vi "cam3 analyse.vi"() -> (0 "G3 chiffre":string, 1 "Y4 chiffre":string, 2 "Y7 chiffre":string, 3 "R2 chiffre":string, 4 "R7 chiffre":string, 5 "G6 chiffre":string, 7 "G9 chiffre":string, 9 "Y1 chiffre":string, 11 "Y2 chiffre":string, 12 "Y3 chiffre":string, 13 "R1 chiffre":string, 14 "R4 chiffre":string)   [LabVIEW 2019]
uses:
  <vilib>/vision/Classification.llb/IMAQ Classifier Read Options.ctl
  <vilib>/vision/NI_Vision_Development_Module.lvlib
panel:
  in  "R7":T1={"Global Rectangle"=[0, 0, 1279, 959], "Contours"=[{"ID"=enum."External", "Type"=3, "Coordinates"=[0, 0, 1279, 959]}]} {"Contours"."Type" items=["No Selection", "Point", "Line", "Rectangle", "Oval", "Polygon", "Freehand Region", "Annulus", "Unused2", "Unused3", "Broken Line", "Freehand Line", "Rotated Rectangle"]}
  out "R7":string[](array[string])
  in  "Y4   3":T1={"Global Rectangle"=[0, 0, 1279, 959], "Contours"=[{"ID"=enum."External", "Type"=3, "Coordinates"=[0, 0, 1279, 959]}]} {"Contours"."Type" items=["No Selection", "Point", "Line", "Rectangle", "Oval", "Polygon", "Freehand Region", "Annulus", "Unused2", "Unused3", "Broken Line", "Freehand Line", "Rotated Rectangle"]}
  out "Y4 2":string[](array[string])
  in  "error in":errorcluster
  out "Coordinates":i32[](array[numeric])
  in  "R4":T1={"Global Rectangle"=[0, 0, 1279, 959], "Contours"=[{"ID"=enum."External", "Type"=3, "Coordinates"=[0, 0, 1279, 959]}]} {"Contours"."Type" items=["No Selection", "Point", "Line", "Rectangle", "Oval", "Polygon", "Freehand Region", "Annulus", "Unused2", "Unused3", "Broken Line", "Freehand Line", "Rotated Rectangle"]}
  out "R4":string[](array[string])
  in  "R2":T1={"Global Rectangle"=[0, 0, 1279, 959], "Contours"=[{"ID"=enum."External", "Type"=3, "Coordinates"=[0, 0, 1279, 959]}]} {"Contours"."Type" items=["No Selection", "Point", "Line", "Rectangle", "Oval", "Polygon", "Freehand Region", "Annulus", "Unused2", "Unused3", "Broken Line", "Freehand Line", "Rotated Rectangle"]}
  out "R2":string[](array[string])
  in  "R1":T1={"Global Rectangle"=[0, 0, 1279, 959], "Contours"=[{"ID"=enum."External", "Type"=3, "Coordinates"=[0, 0, 1279, 959]}]} {"Contours"."Type" items=["No Selection", "Point", "Line", "Rectangle", "Oval", "Polygon", "Freehand Region", "Annulus", "Unused2", "Unused3", "Broken Line", "Freehand Line", "Rotated Rectangle"]}
  out "R1":string[](array[string])
  in  "Y7":T1={"Global Rectangle"=[0, 0, 1279, 959], "Contours"=[{"ID"=enum."External", "Type"=3, "Coordinates"=[0, 0, 1279, 959]}]} {"Contours"."Type" items=["No Selection", "Point", "Line", "Rectangle", "Oval", "Polygon", "Freehand Region", "Annulus", "Unused2", "Unused3", "Broken Line", "Freehand Line", "Rotated Rectangle"]}
  out "Y7":string[](array[string])
  in  "Y3":T1={"Global Rectangle"=[0, 0, 1279, 959], "Contours"=[{"ID"=enum."External", "Type"=3, "Coordinates"=[0, 0, 1279, 959]}]} {"Contours"."Type" items=["No Selection", "Point", "Line", "Rectangle", "Oval", "Polygon", "Freehand Region", "Annulus", "Unused2", "Unused3", "Broken Line", "Freehand Line", "Rotated Rectangle"]}
  out "Y3":string[](array[string])
  in  "Y2":T1={"Global Rectangle"=[0, 0, 1279, 959], "Contours"=[{"ID"=enum."External", "Type"=3, "Coordinates"=[0, 0, 1279, 959]}]} {"Contours"."Type" items=["No Selection", "Point", "Line", "Rectangle", "Oval", "Polygon", "Freehand Region", "Annulus", "Unused2", "Unused3", "Broken Line", "Freehand Line", "Rotated Rectangle"]}
  out "Y2":string[](array[string])
  in  "Y1":T1={"Global Rectangle"=[0, 0, 1279, 959], "Contours"=[{"ID"=enum."External", "Type"=3, "Coordinates"=[0, 0, 1279, 959]}]} {"Contours"."Type" items=["No Selection", "Point", "Line", "Rectangle", "Oval", "Polygon", "Freehand Region", "Annulus", "Unused2", "Unused3", "Broken Line", "Freehand Line", "Rotated Rectangle"]}
  out "Y1":string[](array[string])
  in  "G9":T1={"Global Rectangle"=[0, 0, 1279, 959], "Contours"=[{"ID"=enum."External", "Type"=3, "Coordinates"=[0, 0, 1279, 959]}]} {"Contours"."Type" items=["No Selection", "Point", "Line", "Rectangle", "Oval", "Polygon", "Freehand Region", "Annulus", "Unused2", "Unused3", "Broken Line", "Freehand Line", "Rotated Rectangle"]}
  out "G9":string[](array[string])
  in  "G6":T1={"Global Rectangle"=[0, 0, 1279, 959], "Contours"=[{"ID"=enum."External", "Type"=3, "Coordinates"=[0, 0, 1279, 959]}]} {"Contours"."Type" items=["No Selection", "Point", "Line", "Rectangle", "Oval", "Polygon", "Freehand Region", "Annulus", "Unused2", "Unused3", "Broken Line", "Freehand Line", "Rotated Rectangle"]}
  out "G6":string[](array[string])
  in  "G3":T1={"Global Rectangle"=[640, 450, 686, 504], "Contours"=[{"ID"=enum."External", "Type"=3, "Coordinates"=[640, 450, 686, 504]}]} {"Contours"."Type" items=["No Selection", "Point", "Line", "Rectangle", "Oval", "Polygon", "Freehand Region", "Annulus", "Unused2", "Unused3", "Broken Line", "Freehand Line", "Rotated Rectangle"]}
  out "Image Out 2":T2(plugin-control)
  out "G3":string[](array[string])
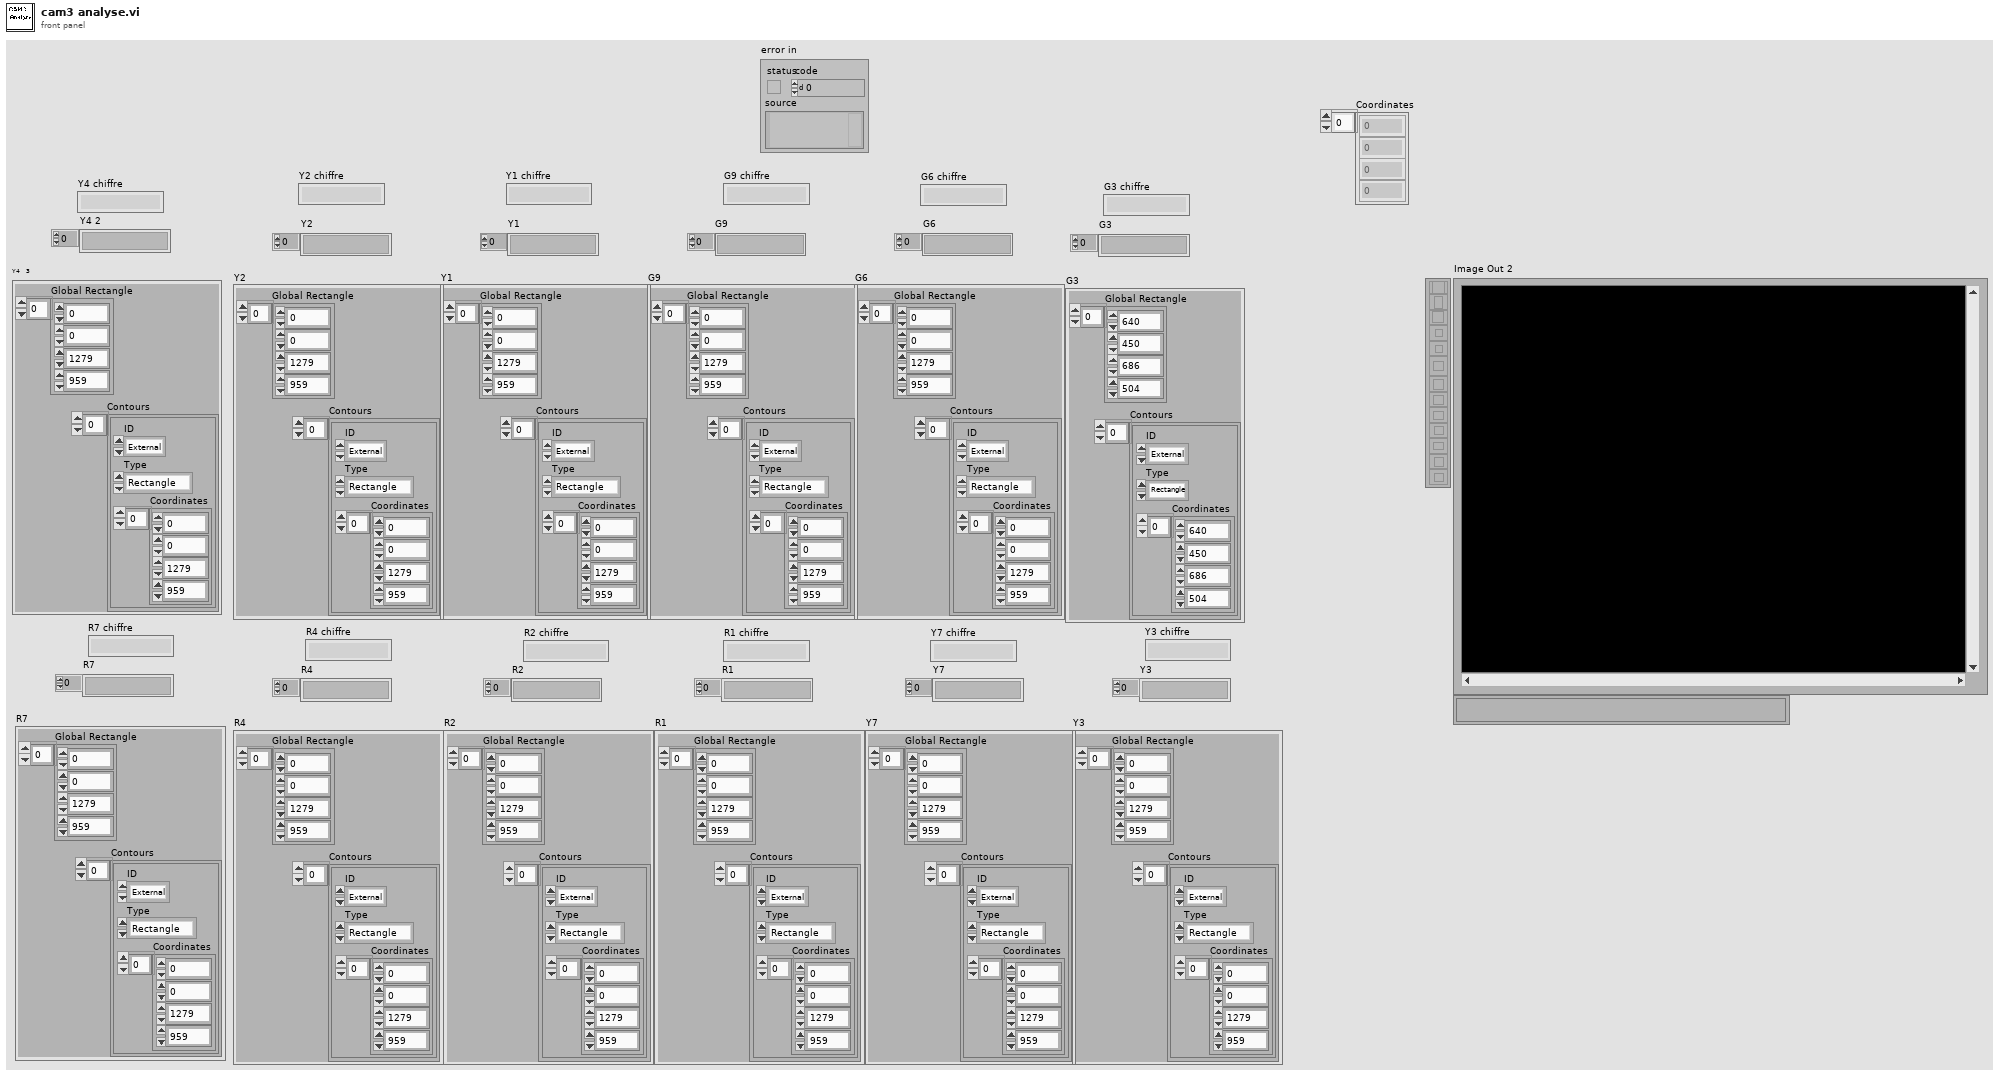
[diagram p1: front panel]
types:
  T1 = cluster{"Global Rectangle":i32[], "Contours":cluster{"ID":enum32{"External", "Internal"}, "Type":u32, "Coordinates":i32[]}[]}
  T2 = typedef "IMAQ Image.ctl" = refnum<image>
  T3 = typedef "IMAQ Classifier Read Options.ctl" = i32
  T4 = typedef "IMAQ Classifier Session.ctl" = refnum<k1>
  T5 = typedef "ROI Descriptor" = cluster{"Global Rectangle":i32[], "Contours":cluster{"ID":enum32{"External", "Internal"}, "Type":u32, "Coordinates":i32[]}[]}
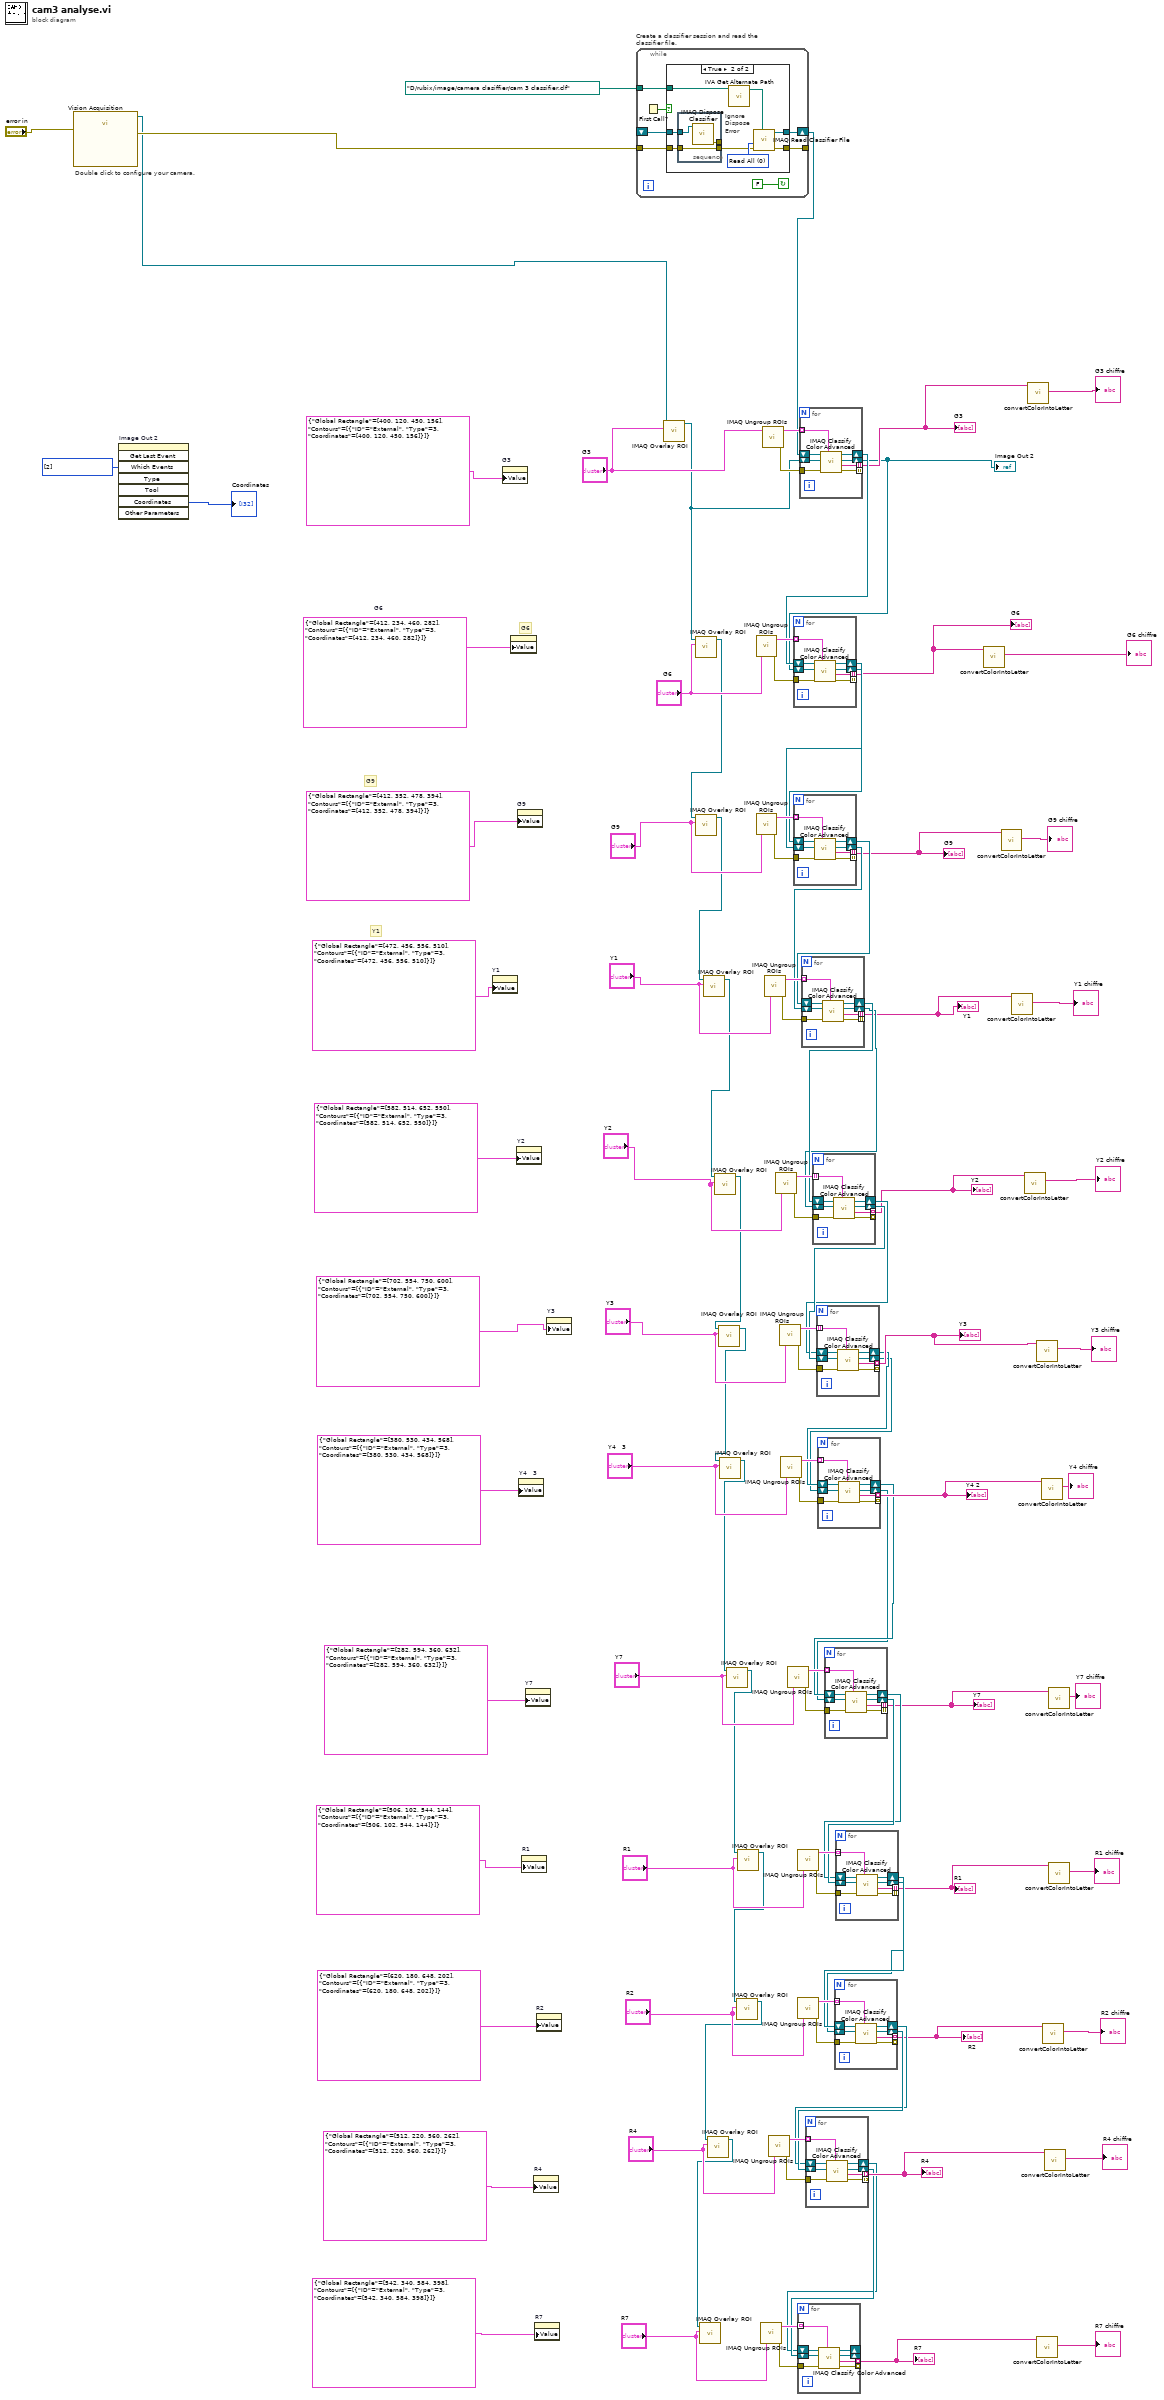
[diagram p0: block diagram]
diagram:
  w27 = i32[] [2] items=["No Event"=0, "Click Event"=1, "Draw Event"=2, "Size Event"=4, "Scroll Event"=5, "Double Click Event"=8] ("Which Events")
  # "G6"
  # "Y1"
  # "G9"
  # "Double click to configure your camera."
  n1 = call "Vision Acquisition"("error in"="error in") -> ("Image Out"=w24:T2, "error out"=w112:errorcluster)  [unwired: 25 in]
  n2 = invoke on="Image Out 2" class="ImageControl" method="Get Last Event"("Which Events"=w27) -> ("Coordinates"=→"Coordinates":i32[])  [unwired: 7 in, 7 out]
  n3 = property on="Y1" class="Clust (strict)"("Value"=T1 {"Global Rectangle"=[472, 456, 556, 510], "Contours"=[{"ID"=enum."External", "Type"=3, "Coordinates"=[472, 456, 556, 510]}]} ("ROI Descriptor (Color Classification 1)")) -> ()  [unwired: 2 in, 2 out]
  n4 = property on="G3" class="Clust (strict)"("Value"=T1 {"Global Rectangle"=[400, 120, 450, 156], "Contours"=[{"ID"=enum."External", "Type"=3, "Coordinates"=[400, 120, 450, 156]}]} ("ROI Descriptor (Color Classification 1)")) -> ()  [unwired: 2 in, 2 out]
  n5 = property on="G6" class="Clust (strict)"("Value"=T1 {"Global Rectangle"=[412, 234, 460, 282], "Contours"=[{"ID"=enum."External", "Type"=3, "Coordinates"=[412, 234, 460, 282]}]} ("ROI Descriptor (Color Classification 1)")) -> ()  [unwired: 2 in, 2 out]
  n6 = property on="Y2" class="Clust (strict)"("Value"=T1 {"Global Rectangle"=[582, 514, 652, 550], "Contours"=[{"ID"=enum."External", "Type"=3, "Coordinates"=[582, 514, 652, 550]}]} ("ROI Descriptor (Color Classification 1)")) -> ()  [unwired: 2 in, 2 out]
  n7 = property on="G9" class="Clust (strict)"("Value"=T1 {"Global Rectangle"=[412, 352, 478, 394], "Contours"=[{"ID"=enum."External", "Type"=3, "Coordinates"=[412, 352, 478, 394]}]} ("ROI Descriptor (Color Classification 1)")) -> ()  [unwired: 2 in, 2 out]
  n8 = property on="Y4   3" class="Clust (strict)"("Value"=T1 {"Global Rectangle"=[380, 530, 434, 568], "Contours"=[{"ID"=enum."External", "Type"=3, "Coordinates"=[380, 530, 434, 568]}]} ("ROI Descriptor (Color Classification 1)")) -> ()  [unwired: 2 in, 2 out]
  n9 = property on="R1" class="Clust (strict)"("Value"=T1 {"Global Rectangle"=[506, 102, 544, 144], "Contours"=[{"ID"=enum."External", "Type"=3, "Coordinates"=[506, 102, 544, 144]}]} ("ROI Descriptor (Color Classification 1)")) -> ()  [unwired: 2 in, 2 out]
  n10 = property on="Y7" class="Clust (strict)"("Value"=T1 {"Global Rectangle"=[282, 594, 360, 632], "Contours"=[{"ID"=enum."External", "Type"=3, "Coordinates"=[282, 594, 360, 632]}]} ("ROI Descriptor (Color Classification 1)")) -> ()  [unwired: 2 in, 2 out]
  n11 = property on="R4" class="Clust (strict)"("Value"=T1 {"Global Rectangle"=[512, 220, 560, 262], "Contours"=[{"ID"=enum."External", "Type"=3, "Coordinates"=[512, 220, 560, 262]}]} ("ROI Descriptor (Color Classification 1)")) -> ()  [unwired: 2 in, 2 out]
  n12 = property on="R7" class="Clust (strict)"("Value"=T1 {"Global Rectangle"=[542, 340, 584, 398], "Contours"=[{"ID"=enum."External", "Type"=3, "Coordinates"=[542, 340, 584, 398]}]} ("ROI Descriptor (Color Classification 1)")) -> ()  [unwired: 2 in, 2 out]
  n13 = property on="R2" class="Clust (strict)"("Value"=T1 {"Global Rectangle"=[620, 180, 648, 202], "Contours"=[{"ID"=enum."External", "Type"=3, "Coordinates"=[620, 180, 648, 202]}]} ("ROI Descriptor (Color Classification 1)")) -> ()  [unwired: 2 in, 2 out]
  n14 = property on="Y3" class="Clust (strict)"("Value"=T1 {"Global Rectangle"=[702, 554, 750, 600], "Contours"=[{"ID"=enum."External", "Type"=3, "Coordinates"=[702, 554, 750, 600]}]} ("ROI Descriptor (Color Classification 1)")) -> ()  [unwired: 2 in, 2 out]
  n15 = while "Create a classifier session and read the classifier file." {
    shift-right: [w119] -> w23
    shift-left: _ -> [w118]
    tunnel: w112 -> [w116]
    tunnel: [w115] -> _
    tunnel: path "D:/rubix/image/camera clasiffier/cam 3 classifier.clf" ("File Path") -> [w114]
    stop <- FALSE continue-if-true
    n16 = First Call?() -> (First Call?: T/F=w113:bool)
    n17 = case shown="True" w113 {
      tunnel: [w121 w128] -> w119
      tunnel: w118 -> [w121 w126]
      tunnel: w116 -> [w120 w125]
      tunnel: [w120 w127] -> w115
      tunnel: w114 -> [_ w123]
      frame False {
      }
      frame True {
        w129 = T3 0 items=["Read All", "Add Samples, Do Not Change Options", "Read Options, Do Not Add Samples"] ("Read Options")
        # "Ignore Dispose Error"
        n18 = stacked-sequence {
          tunnel: w126 -> [w132]
          tunnel: w125 -> [w131]
          tunnel: [w131] -> w124
          tunnel: [w130] -> _
          frame #0 {
            n19 = call "IMAQ Dispose Classifier"("Classifier Session"=w132) -> ("error out"=w130:errorcluster)  [unwired: 1 in, 9 out]
          }
        }
        n20 = call <vilib>:"IVA Get Alternate Path.vi"("Path In"=w123) -> ("Path Out"=w122:path)  [unwired: 10 out]
        n21 = call "IMAQ Read Classifier File"("File Path"=w122, "error in (no error)"=w124, "Read Options"=w129) -> ("error out"=w127:errorcluster, "Classifier Session"=w128:T4)  [unwired: 1 in, 6 out]
      }
    }
  }
  n22 = call "IMAQ Overlay ROI"("ROI Descriptor"="G3", "Image"=w24) -> ("Image Out"=w26:T2)  [unwired: 8 in, 1 out]
  n23 = call "IMAQ Overlay ROI"("ROI Descriptor"="G6", "Image"=w26) -> ("Image Out"=w102:T2)  [unwired: 8 in, 1 out]
  n24 = call "IMAQ Overlay ROI"("ROI Descriptor"="G9", "Image"=w102) -> ("Image Out"=w94:T2)  [unwired: 8 in, 1 out]
  n25 = call "IMAQ Overlay ROI"("ROI Descriptor"="Y1", "Image"=w94) -> ("Image Out"=w86:T2)  [unwired: 8 in, 1 out]
  n26 = call "IMAQ Overlay ROI"("ROI Descriptor"="Y2", "Image"=w86) -> ("Image Out"=w79:T2)  [unwired: 8 in, 1 out]
  n27 = call "IMAQ Overlay ROI"("ROI Descriptor"="Y3", "Image"=w79) -> ("Image Out"=w14:T2)  [unwired: 8 in, 1 out]
  n28 = call "IMAQ Overlay ROI"("ROI Descriptor"="Y4   3", "Image"=w14) -> ("Image Out"=w15:T2)  [unwired: 8 in, 1 out]
  n29 = call "IMAQ Overlay ROI"("ROI Descriptor"="Y7", "Image"=w15) -> ("Image Out"=w70:T2)  [unwired: 8 in, 1 out]
  n30 = call "IMAQ Overlay ROI"("ROI Descriptor"="R1", "Image"=w70) -> ("Image Out"=w60:T2)  [unwired: 8 in, 1 out]
  n31 = call "IMAQ Overlay ROI"("ROI Descriptor"="R2", "Image"=w60) -> ("Image Out"=w56:T2)  [unwired: 8 in, 1 out]
  n32 = call "IMAQ Overlay ROI"("ROI Descriptor"="R4", "Image"=w56) -> ("Image Out"=w1:T2)  [unwired: 8 in, 1 out]
  n33 = call "IMAQ Overlay ROI"("ROI Descriptor"="R7", "Image"=w1) -> ()  [unwired: 8 in, 2 out]
  n34 = call "IMAQ Ungroup ROIs"("ROI Descriptor"="G6") -> ("error out"=w108:errorcluster, "ROI Descriptors out"=w107:T5[])  [unwired: 1 in, 2 out]
  n35 = call "IMAQ Ungroup ROIs"("ROI Descriptor"="G9") -> ("error out"=w104:errorcluster, "ROI Descriptors out"=w103:T5[])  [unwired: 1 in, 2 out]
  n36 = call "IMAQ Ungroup ROIs"("ROI Descriptor"="R7") -> ("error out"=w9:errorcluster, "ROI Descriptors out"=w8:T5[])  [unwired: 1 in, 2 out]
  n37 = call "IMAQ Ungroup ROIs"("ROI Descriptor"="G3") -> ("error out"=w110:errorcluster, "ROI Descriptors out"=w109:T5[])  [unwired: 1 in, 2 out]
  n38 = call "IMAQ Ungroup ROIs"("ROI Descriptor"="Y1") -> ("error out"=w97:errorcluster, "ROI Descriptors out"=w96:T5[])  [unwired: 1 in, 2 out]
  n39 = call "IMAQ Ungroup ROIs"("ROI Descriptor"="R4") -> ("error out"=w59:errorcluster, "ROI Descriptors out"=w58:T5[])  [unwired: 1 in, 2 out]
  n40 = call "IMAQ Ungroup ROIs"("ROI Descriptor"="Y2") -> ("error out"=w90:errorcluster, "ROI Descriptors out"=w89:T5[])  [unwired: 1 in, 2 out]
  n41 = call "IMAQ Ungroup ROIs"("ROI Descriptor"="Y3") -> ("error out"=w83:errorcluster, "ROI Descriptors out"=w82:T5[])  [unwired: 1 in, 2 out]
  n42 = call "IMAQ Ungroup ROIs"("ROI Descriptor"="Y4   3") -> ("error out"=w21:errorcluster, "ROI Descriptors out"=w20:T5[])  [unwired: 1 in, 2 out]
  n43 = call "IMAQ Ungroup ROIs"("ROI Descriptor"="Y7") -> ("error out"=w77:errorcluster, "ROI Descriptors out"=w76:T5[])  [unwired: 1 in, 2 out]
  n44 = call "IMAQ Ungroup ROIs"("ROI Descriptor"="R2") -> ("error out"=w66:errorcluster, "ROI Descriptors out"=w65:T5[])  [unwired: 1 in, 2 out]
  n45 = call "IMAQ Ungroup ROIs"("ROI Descriptor"="R1") -> ("error out"=w73:errorcluster, "ROI Descriptors out"=w72:T5[])  [unwired: 1 in, 2 out]
  n46 = for {
    tunnel: [w140] -> w33 mode=indexing
    tunnel: [w139] -> _ mode=indexing
    tunnel: w110 -> [w137]
    tunnel: w109 -> [w136] mode=indexing
    shift-right: [w134] -> w25
    shift-left: w26 -> [w135]
    shift-right: [w133] -> w35
    shift-left: w23 -> [w138]
    n47 = call "IMAQ Classify Color Advanced"("ROI Descriptor"=w136, "error in (no error)"=w137, "Image"=w135, "Classifier Session"=w138) -> ("error out"=w139:errorcluster, "Class"=w140:string, "Image (dup)"=w134:T2, "Classifier Session (dup)"=w133:T4)  [unwired: 4 out]
  }
  "G3" <- w33
  "Image Out 2" <- w25
  n48 = for {
    tunnel: [w148] -> w30 mode=indexing
    tunnel: [w147] -> _ mode=indexing
    tunnel: w108 -> [w145]
    tunnel: w107 -> [w144] mode=indexing
    shift-right: [w142] -> w100
    shift-left: w25 -> [w143]
    shift-right: [w141] -> w101
    shift-left: w35 -> [w146]
    n49 = call "IMAQ Classify Color Advanced"("ROI Descriptor"=w144, "error in (no error)"=w145, "Image"=w143, "Classifier Session"=w146) -> ("error out"=w147:errorcluster, "Class"=w148:string, "Image (dup)"=w142:T2, "Classifier Session (dup)"=w141:T4)  [unwired: 4 out]
  }
  "G6" <- w30
  n50 = for {
    tunnel: [w156] -> w51 mode=indexing
    tunnel: [w155] -> _ mode=indexing
    tunnel: w104 -> [w153]
    tunnel: w103 -> [w152] mode=indexing
    shift-right: [w150] -> w93
    shift-left: w100 -> [w151]
    shift-right: [w149] -> w92
    shift-left: w101 -> [w154]
    n51 = call "IMAQ Classify Color Advanced"("ROI Descriptor"=w152, "error in (no error)"=w153, "Image"=w151, "Classifier Session"=w154) -> ("error out"=w155:errorcluster, "Class"=w156:string, "Image (dup)"=w150:T2, "Classifier Session (dup)"=w149:T4)  [unwired: 4 out]
  }
  "G9" <- w51
  n52 = for {
    tunnel: [w164] -> w50 mode=indexing
    tunnel: [w163] -> _ mode=indexing
    tunnel: w97 -> [w161]
    tunnel: w96 -> [w160] mode=indexing
    shift-right: [w158] -> w87
    shift-left: w93 -> [w159]
    shift-right: [w157] -> w88
    shift-left: w92 -> [w162]
    n53 = call "IMAQ Classify Color Advanced"("ROI Descriptor"=w160, "error in (no error)"=w161, "Image"=w159, "Classifier Session"=w162) -> ("error out"=w163:errorcluster, "Class"=w164:string, "Image (dup)"=w158:T2, "Classifier Session (dup)"=w157:T4)  [unwired: 4 out]
  }
  "Y1" <- w50
  n54 = for {
    tunnel: [w172] -> w49 mode=indexing
    tunnel: [w171] -> _ mode=indexing
    tunnel: w90 -> [w169]
    tunnel: w89 -> [w168] mode=indexing
    shift-right: [w166] -> w81
    shift-left: w87 -> [w167]
    shift-right: [w165] -> w80
    shift-left: w88 -> [w170]
    n55 = call "IMAQ Classify Color Advanced"("ROI Descriptor"=w168, "error in (no error)"=w169, "Image"=w167, "Classifier Session"=w170) -> ("error out"=w171:errorcluster, "Class"=w172:string, "Image (dup)"=w166:T2, "Classifier Session (dup)"=w165:T4)  [unwired: 4 out]
  }
  "Y2" <- w49
  n56 = for {
    tunnel: [w180] -> w48 mode=indexing
    tunnel: [w179] -> _ mode=indexing
    tunnel: w83 -> [w177]
    tunnel: w82 -> [w176] mode=indexing
    shift-right: [w174] -> w12
    shift-left: w81 -> [w175]
    shift-right: [w173] -> w13
    shift-left: w80 -> [w178]
    n57 = call "IMAQ Classify Color Advanced"("ROI Descriptor"=w176, "error in (no error)"=w177, "Image"=w175, "Classifier Session"=w178) -> ("error out"=w179:errorcluster, "Class"=w180:string, "Image (dup)"=w174:T2, "Classifier Session (dup)"=w173:T4)  [unwired: 4 out]
  }
  "Y3" <- w48
  n58 = for {
    tunnel: [w188] -> w17 mode=indexing
    tunnel: [w187] -> _ mode=indexing
    tunnel: w21 -> [w185]
    tunnel: w20 -> [w184] mode=indexing
    shift-right: [w182] -> w10
    shift-left: w12 -> [w183]
    shift-right: [w181] -> w11
    shift-left: w13 -> [w186]
    n59 = call "IMAQ Classify Color Advanced"("ROI Descriptor"=w184, "error in (no error)"=w185, "Image"=w183, "Classifier Session"=w186) -> ("error out"=w187:errorcluster, "Class"=w188:string, "Image (dup)"=w182:T2, "Classifier Session (dup)"=w181:T4)  [unwired: 4 out]
  }
  "Y4 2" <- w17
  n60 = for {
    tunnel: [w196] -> w47 mode=indexing
    tunnel: [w195] -> _ mode=indexing
    tunnel: w77 -> [w193]
    tunnel: w76 -> [w192] mode=indexing
    shift-right: [w190] -> w69
    shift-left: w10 -> [w191]
    shift-right: [w189] -> w68
    shift-left: w11 -> [w194]
    n61 = call "IMAQ Classify Color Advanced"("ROI Descriptor"=w192, "error in (no error)"=w193, "Image"=w191, "Classifier Session"=w194) -> ("error out"=w195:errorcluster, "Class"=w196:string, "Image (dup)"=w190:T2, "Classifier Session (dup)"=w189:T4)  [unwired: 4 out]
  }
  "Y7" <- w47
  n62 = for {
    tunnel: [w204] -> w46 mode=indexing
    tunnel: [w203] -> _ mode=indexing
    tunnel: w73 -> [w201]
    tunnel: w72 -> [w200] mode=indexing
    shift-right: [w198] -> w63
    shift-left: w69 -> [w199]
    shift-right: [w197] -> w64
    shift-left: w68 -> [w202]
    n63 = call "IMAQ Classify Color Advanced"("ROI Descriptor"=w200, "error in (no error)"=w201, "Image"=w199, "Classifier Session"=w202) -> ("error out"=w203:errorcluster, "Class"=w204:string, "Image (dup)"=w198:T2, "Classifier Session (dup)"=w197:T4)  [unwired: 4 out]
  }
  "R1" <- w46
  n64 = for {
    tunnel: [w212] -> w45 mode=indexing
    tunnel: [w211] -> _ mode=indexing
    tunnel: w66 -> [w209]
    tunnel: w65 -> [w208] mode=indexing
    shift-right: [w206] -> w55
    shift-left: w63 -> [w207]
    shift-right: [w205] -> w54
    shift-left: w64 -> [w210]
    n65 = call "IMAQ Classify Color Advanced"("ROI Descriptor"=w208, "error in (no error)"=w209, "Image"=w207, "Classifier Session"=w210) -> ("error out"=w211:errorcluster, "Class"=w212:string, "Image (dup)"=w206:T2, "Classifier Session (dup)"=w205:T4)  [unwired: 4 out]
  }
  "R2" <- w45
  n66 = for {
    tunnel: [w220] -> w44 mode=indexing
    tunnel: [w219] -> _ mode=indexing
    tunnel: w59 -> [w217]
    tunnel: w58 -> [w216] mode=indexing
    shift-right: [w214] -> w3
    shift-left: w55 -> [w215]
    shift-right: [w213] -> w2
    shift-left: w54 -> [w218]
    n67 = call "IMAQ Classify Color Advanced"("ROI Descriptor"=w216, "error in (no error)"=w217, "Image"=w215, "Classifier Session"=w218) -> ("error out"=w219:errorcluster, "Class"=w220:string, "Image (dup)"=w214:T2, "Classifier Session (dup)"=w213:T4)  [unwired: 4 out]
  }
  "R4" <- w44
  n68 = for {
    tunnel: [w228] -> w6 mode=indexing
    tunnel: [w227] -> _ mode=indexing
    tunnel: w9 -> [w225]
    tunnel: w8 -> [w224] mode=indexing
    shift-right: [w222] -> _
    shift-left: w3 -> [w223]
    shift-right: [w221] -> _
    shift-left: w2 -> [w226]
    n69 = call "IMAQ Classify Color Advanced"("ROI Descriptor"=w224, "error in (no error)"=w225, "Image"=w223, "Classifier Session"=w226) -> ("error out"=w227:errorcluster, "Class"=w228:string, "Image (dup)"=w222:T2, "Classifier Session (dup)"=w221:T4)  [unwired: 4 out]
  }
  "R7" <- w6
  n70 = call "convertColorIntoLetter.vi"("Array"=w30) -> ("String"=→"G6 chiffre":string)  [unwired: 10 in]
  n71 = call "convertColorIntoLetter.vi"("Array"=w51) -> ("String"=→"G9 chiffre":string)  [unwired: 10 in]
  n72 = call "convertColorIntoLetter.vi"("Array"=w50) -> ("String"=→"Y1 chiffre":string)  [unwired: 10 in]
  n73 = call "convertColorIntoLetter.vi"("Array"=w49) -> ("String"=→"Y2 chiffre":string)  [unwired: 10 in]
  n74 = call "convertColorIntoLetter.vi"("Array"=w33) -> ("String"=→"G3 chiffre":string)  [unwired: 10 in]
  n75 = call "convertColorIntoLetter.vi"("Array"=w48) -> ("String"=→"Y3 chiffre":string)  [unwired: 10 in]
  n76 = call "convertColorIntoLetter.vi"("Array"=w6) -> ("String"=→"R7 chiffre":string)  [unwired: 10 in]
  n77 = call "convertColorIntoLetter.vi"("Array"=w17) -> ("String"=→"Y4 chiffre":string)  [unwired: 10 in]
  n78 = call "convertColorIntoLetter.vi"("Array"=w45) -> ("String"=→"R2 chiffre":string)  [unwired: 10 in]
  n79 = call "convertColorIntoLetter.vi"("Array"=w44) -> ("String"=→"R4 chiffre":string)  [unwired: 10 in]
  n80 = call "convertColorIntoLetter.vi"("Array"=w47) -> ("String"=→"Y7 chiffre":string)  [unwired: 10 in]
  n81 = call "convertColorIntoLetter.vi"("Array"=w46) -> ("String"=→"R1 chiffre":string)  [unwired: 10 in]
